vi "Generate Partially Closed Signal.vi"(7 "Avg % Open":dbl=1.0 format="%#_13g", 8 "Repetitions":u32=5, 9 "+/- % Open":dbl=90.0 format="%#_13g", 10 "Frequency[Hz]":dbl=5.0 format="%#_13g") -> (0 "Total # of Frequency Samples":i32, 1 "Digital Waveform Graph":digitalwaveform(graph), 2 "CO Frequency":cluster{"duty cycle":dbl, "frequency":dbl}[](array[cluster]), 3 "dt":dbl, 4 "Total # of Digital Samples":i32)   [LabVIEW 2017]
uses:
  <vilib>/Waveform/DTblOps.llb/DTbl Boolean Array to Digital.vi
panel:
  out "Unsigned Frequency Array 2-way":dbl[](graph)
  out "Direction Array 2-way":bool[](array[boolean])
  out "Signed Frequency Array 2-way":dbl[](graph)
  out "Waveform Graph 3":dbl[](graph)
  out "Numeric 2":i32
  out "XY Graph":cluster{dbl[], dbl[]}(graph)
  out "Negative Frequency Array 1-way":dbl[](graph)
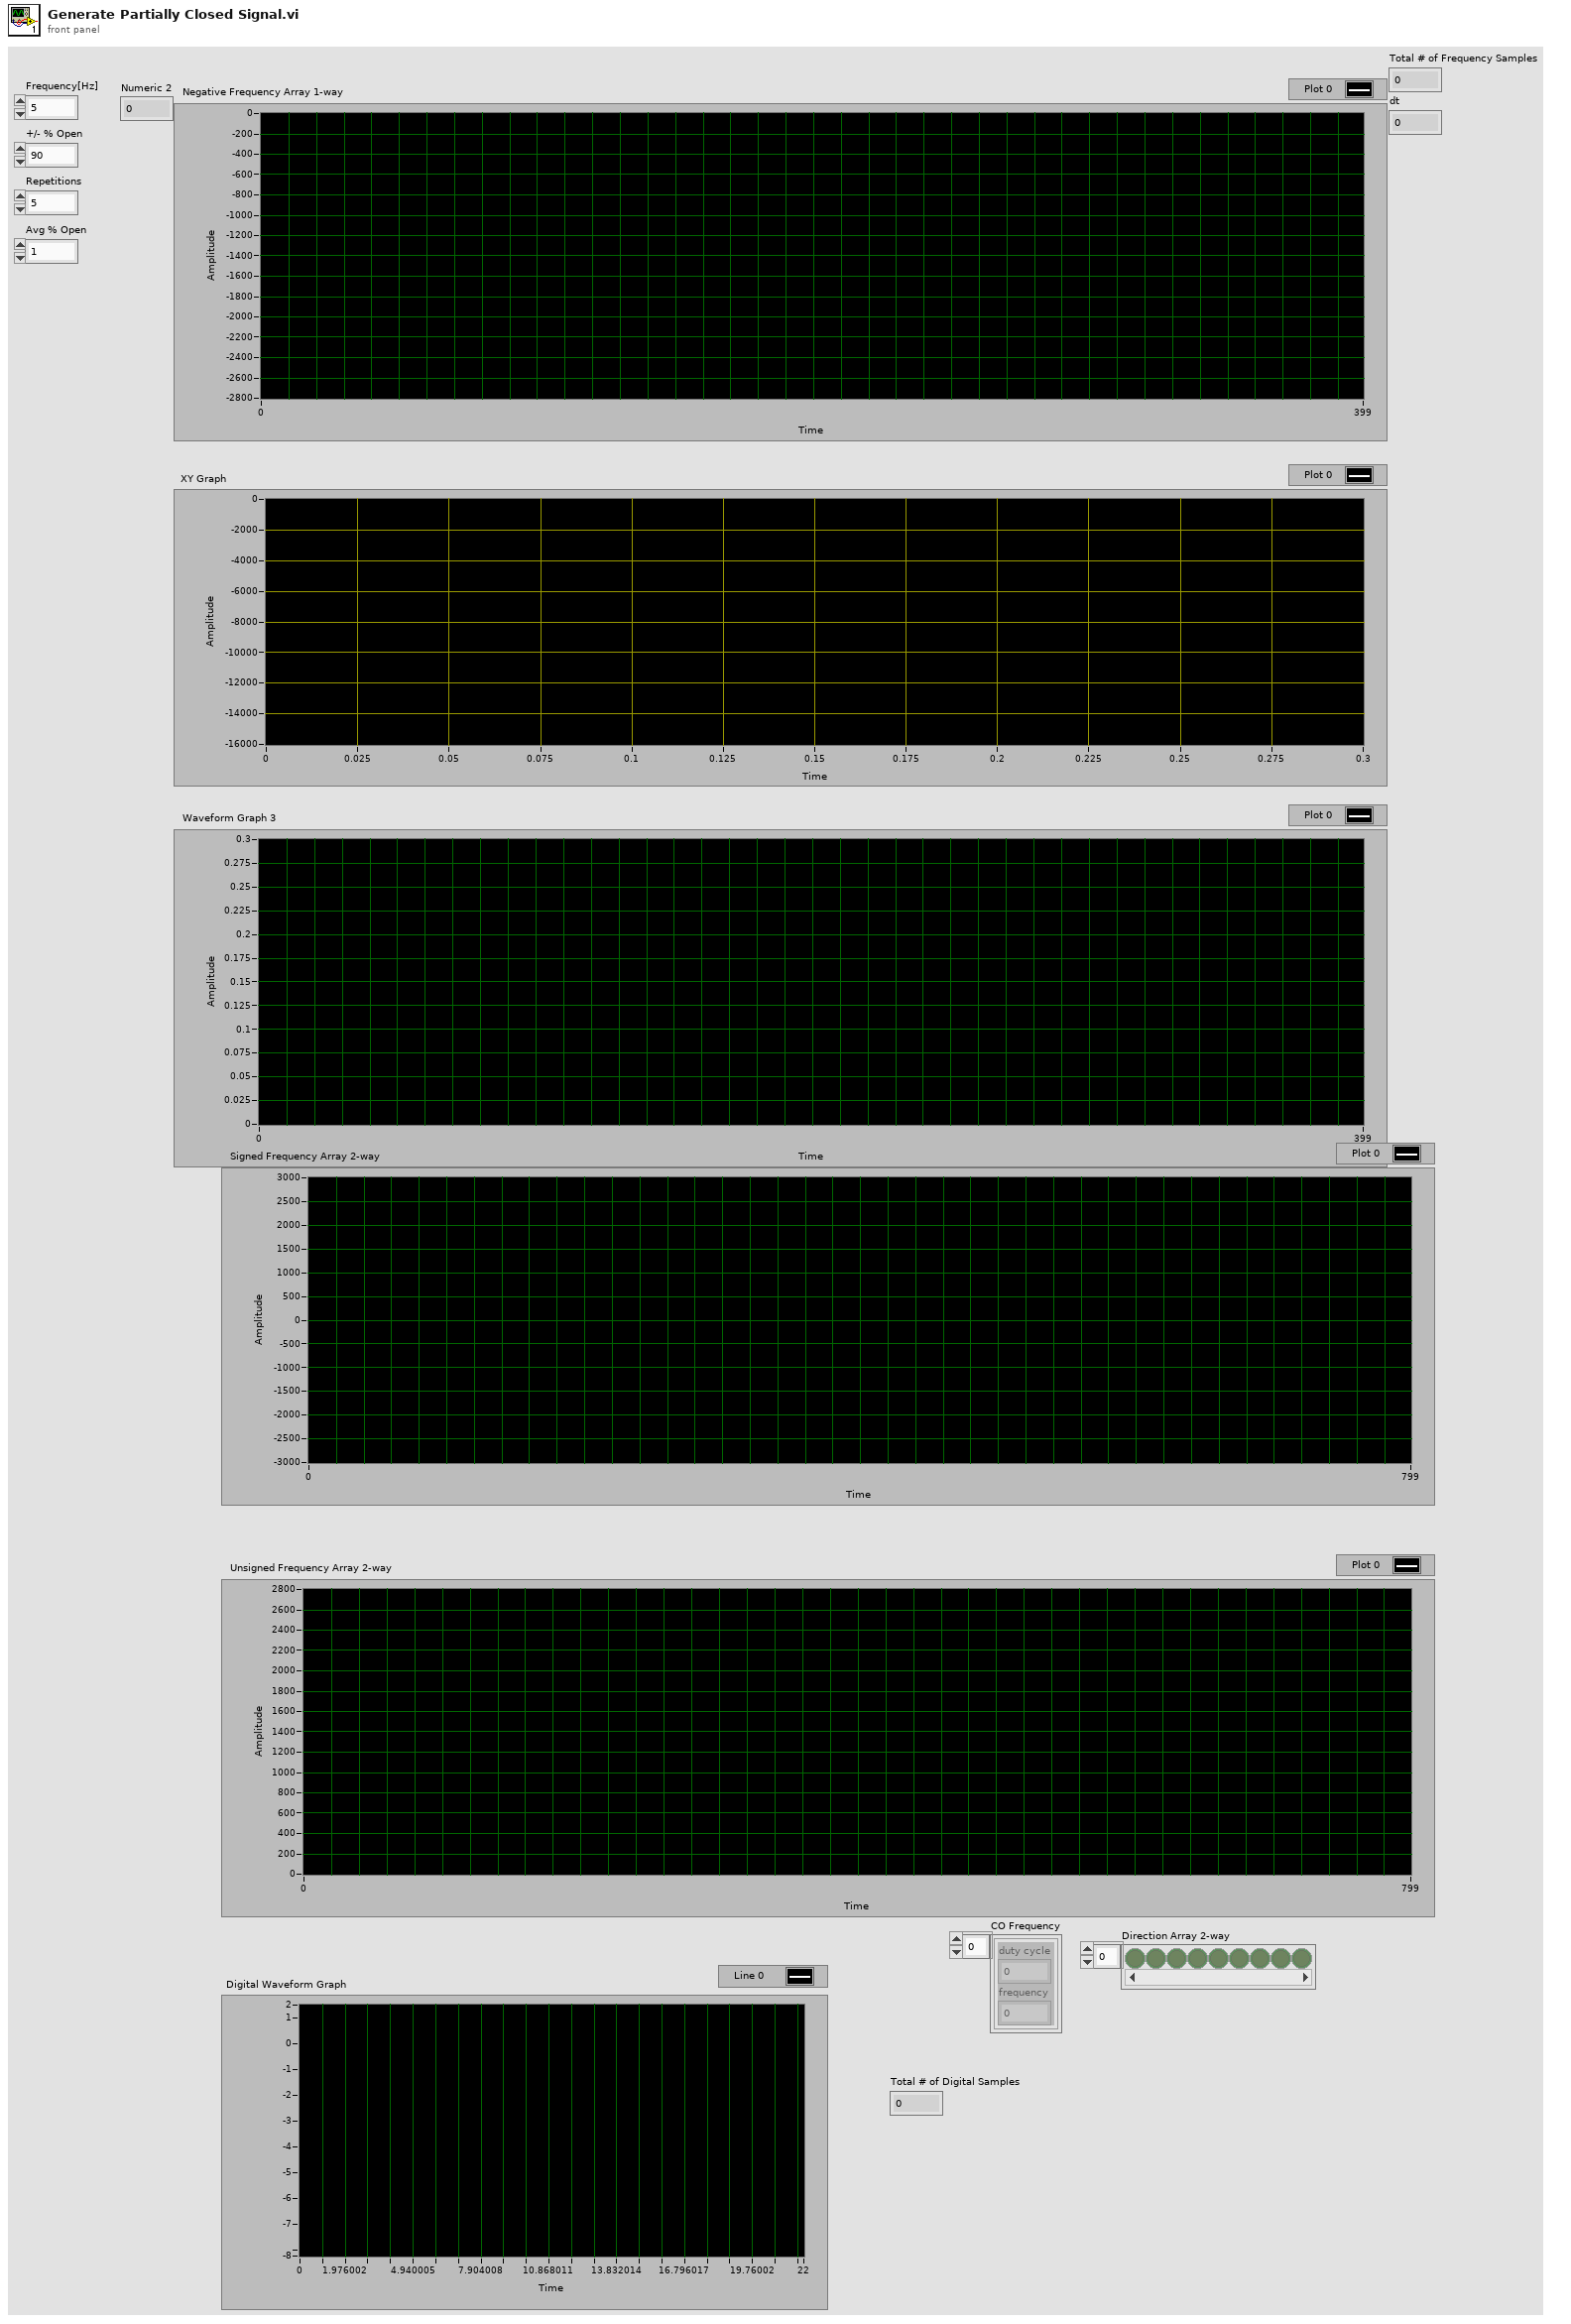
[diagram p1: front panel]
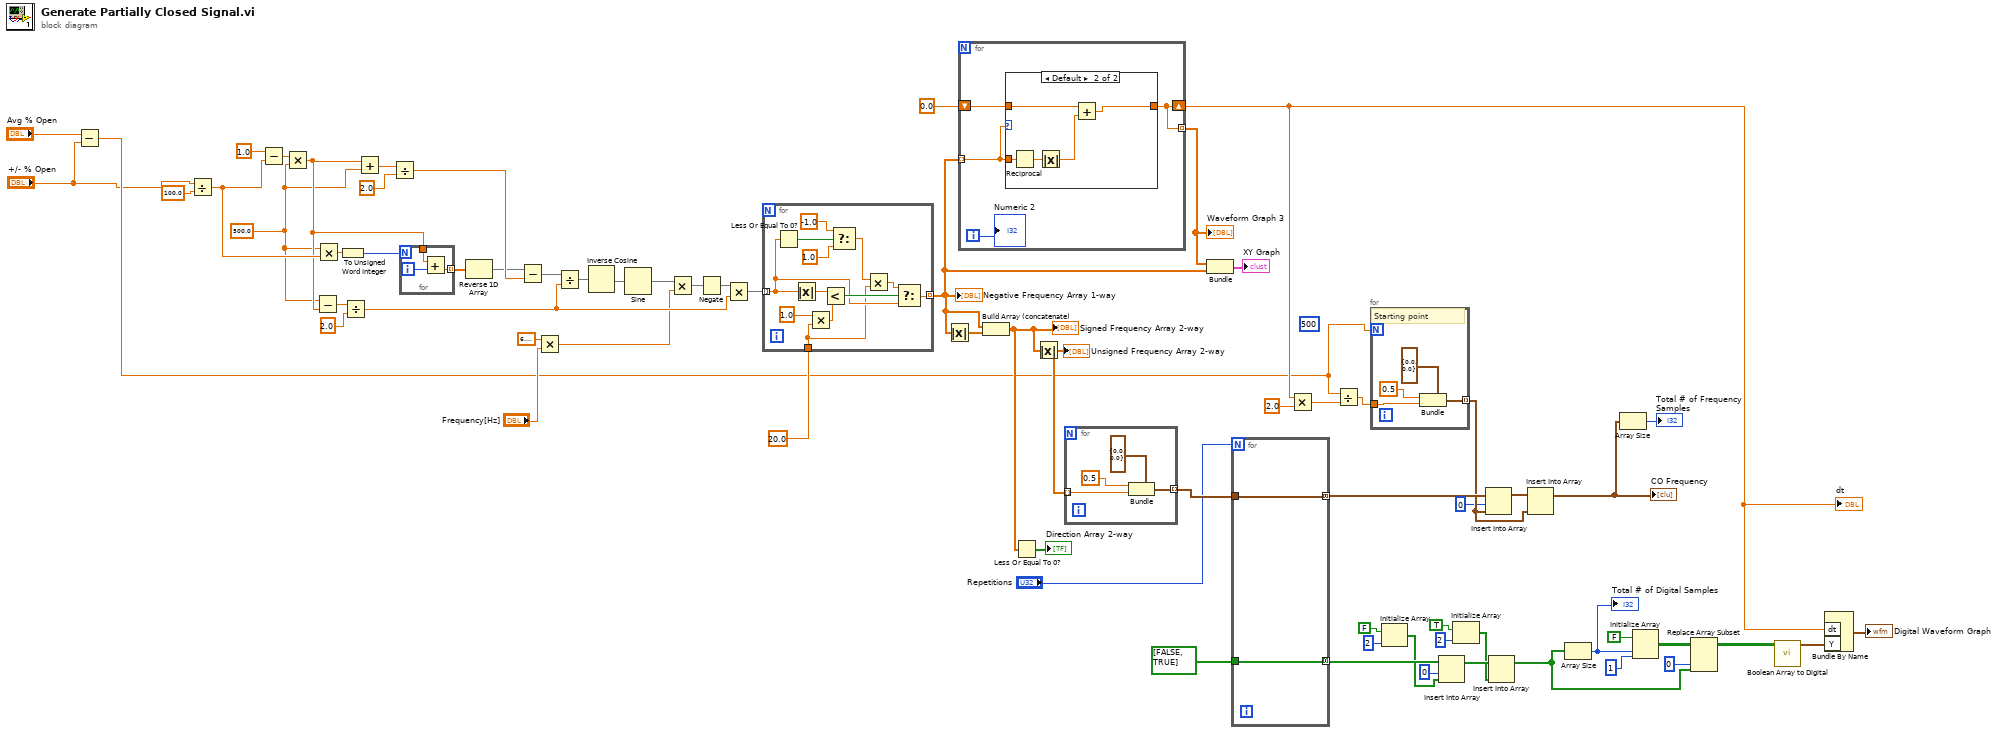
[diagram p0: block diagram]
diagram:
  (unwired) 500
  w5 = 500.0
  n1 = Subtract(x="Avg % Open", y="+/- % Open") -> (x-y=w2:dbl)
  n2 = Divide(x="+/- % Open", y=100.0) -> (x/y=w67:dbl)
  n3 = Subtract(x=1.0, y=w67) -> (x-y=w68:dbl)
  n4 = Multiply(x=w68, y=w5) -> (x*y=w55:dbl)
  n5 = Subtract(x=w5, y=w55) -> (x-y=w54:dbl)
  n6 = Multiply(x=w5, y=w67) -> (x*y=w66:dbl)
  n7 = To Unsigned Word Integer(number=w66) -> (unsigned 16bit integer=w40:u16)
  n8 = Divide(x=w54, y=2.0) -> (x/y=w52:dbl)
  n9 = Add(x=w55, y=w5) -> (x+y=w64:dbl)
  n10 = Divide(x=w64, y=2.0) -> (x/y=w62:dbl)
  n11 = for {
    N: w40 -> [_]
    tunnel: [w71] -> w48 mode=indexing
    tunnel: w55 -> [w70]
    i -> [w72]
    n12 = Add(x=w70, y=w72) -> (x+y=w71:dbl)
  }
  n13 = Reverse 1D Array(array=w48) -> (reversed array=w47:dbl[])
  n14 = Subtract(x=w47, y=w62) -> (x-y=w61:dbl[])
  n15 = Multiply(x=6.283185307179586, y="Frequency[Hz]") -> (x*y=w49:dbl)
  n16 = Divide(x=w61, y=w52) -> (x/y=w60:dbl[])
  n17 = Inverse Cosine(1:w60) -> (0:w46:dbl[])
  n18 = Sine(x=w46) -> (sin(x)=w59:dbl[])
  n19 = Multiply(x=w59, y=w49) -> (x*y=w58:dbl[])
  n20 = Negate(x=w58) -> (-x=w57:dbl[])
  n21 = Multiply(x=w57, y=w52) -> (x*y=w44:dbl[])
  n22 = for {
    tunnel: w44 -> [w81] mode=indexing
    tunnel: [w82] -> w43 mode=indexing
    tunnel: 20.0 ("y") -> [w73]
    n23 = Less Or Equal To 0?(x=w81) -> (x <= 0?=w80:bool)
    n24 = Absolute Value(x=w81) -> (abs(x)=w84:dbl)
    n25 = Multiply(x=1.0 ("y"), y=w73) -> (x*y=w77:dbl)
    n26 = Less?(x=w84, y=w77) -> (x < y?=w83:bool)
    n27 = Select(t=-1.0, s=w80, f=1.0 ("t")) -> (s? t:f=w76:dbl)
    n28 = Multiply(x=w76, y=w73) -> (x*y=w75:dbl)
    n29 = Select(t=w75, s=w83, f=w81) -> (s? t:f=w82:dbl)
  }
  "Negative Frequency Array 1-way" <- w43
  n30 = Absolute Value(x=w43) -> (abs(x)=w42:dbl[])
  n31 = for {
    tunnel: w43 -> [w85] mode=indexing
    shift-right: [w86] -> w23
    shift-left: 0.0 -> [w88]
    tunnel: [w86] -> w45 mode=indexing
    i -> [w87]
    n32 = case shown="Default" w85 {
      tunnel: w88 -> [w89 w94]
      tunnel: [w89 w93] -> w86
      tunnel: w85 -> [_ w92]
      frame 0 {
      }
      frame Default {
        n33 = Reciprocal(x=w92) -> (1/x=w91:dbl)
        n34 = Absolute Value(x=w91) -> (abs(x)=w90:dbl)
        n35 = Add(x=w94, y=w90) -> (x+y=w93:dbl)
      }
    }
    "Numeric 2" <- w87
  }
  "Waveform Graph 3" <- w45
  "dt" <- w23
  n36 = Build Array (concatenate)(w43, w42) -> (w41:dbl[])
  "Signed Frequency Array 2-way" <- w41
  n37 = Less Or Equal To 0?(x=w41) -> (x <= 0?=→"Direction Array 2-way":bool[])
  n38 = Absolute Value(x=w41) -> (abs(x)=w27:dbl[])
  "Unsigned Frequency Array 2-way" <- w27
  n39 = for {
    tunnel: w27 -> [w98] mode=indexing
    tunnel: [w96] -> w32 mode=indexing
    n40 = Bundle(cluster=cluster{"duty cycle":dbl, "frequency":dbl} {"duty cycle"=0.0, "frequency"=0.0}, "duty cycle"=0.5 ("t"), "frequency"=w98) -> (w96:cluster{"duty cycle":dbl, "frequency":dbl})
  }
  n41 = Bundle(w45, w43) -> (→"XY Graph":cluster{dbl[], dbl[]})  [unwired: 1 in]
  n42 = for {
    N: "Repetitions" -> [_]
    tunnel: w32 -> [w100]
    tunnel: [w100] -> w26 mode=concatenating
    tunnel: bool[] [FALSE, TRUE] ("new element/subarray") -> [w99]
    tunnel: [w99] -> w25 mode=concatenating
  }
  n43 = Multiply(x=w23, y=2.0) -> (x*y=w21:dbl)
  n44 = Divide(x=w2, y=w21) -> (x/y=w22:dbl)
  n45 = for {
    N: w2 -> [_]
    tunnel: w22 -> [w104]
    tunnel: [w102] -> w19 mode=indexing
    # "Starting point"
    n46 = Bundle(cluster=cluster{"duty cycle":dbl, "frequency":dbl} {"duty cycle"=0.0, "frequency"=0.0}, "duty cycle"=0.5 ("t"), "frequency"=w104) -> (w102:cluster{"duty cycle":dbl, "frequency":dbl})
  }
  n47 = Initialize Array(FALSE ("t"), 2 ("dimension size")) -> (w12:bool[])
  n48 = Insert Into Array(array=w25, index=0, new element=w12) -> (w11:bool[])
  n49 = Initialize Array(TRUE ("t"), 2 ("dimension size")) -> (w8:bool[])
  n50 = Insert Into Array(array=w26, index=0, new element=w19) -> (w16:cluster{"duty cycle":dbl, "frequency":dbl}[])
  n51 = Insert Into Array(array=w11, new element=w8) -> (w18:bool[])  [unwired: 1 in]
  n52 = Insert Into Array(array=w16, new element=w19) -> (w20:cluster{"duty cycle":dbl, "frequency":dbl}[])  [unwired: 1 in]
  "CO Frequency" <- w20
  n53 = Array Size(array=w18) -> (size(s)=w6:i32)
  "Total # of Digital Samples" <- w6
  n54 = Array Size(array=w20) -> (size(s)=→"Total # of Frequency Samples":i32)
  n55 = Initialize Array(FALSE, w6, 1 ("dimension size")) -> (w37:bool[][])
  n56 = Replace Array Subset(array=w37, new element=w18, index (col)=0 ("index (row)")) -> (w7:bool[][])  [unwired: 1 in]
  n57 = call-poly <vilib>:"Boolean Array to Digital.vi"("boolean array"=w7) -> ("digital data"=w38:digitaldata)  [unwired: 3 in, 7 out]
  n58 = Bundle By Name("dt"=w23, "Y"=w38) -> (→"Digital Waveform Graph":digitalwaveform)  [unwired: 1 in]
